vi "AlliGator Format Script Output.vi"(8 "Error In":errorcluster, 11 "Array of Simulation Outputs":T1[](array[typedef]) {"Simulation & Fit Options & Parameters"."Decay Fit Options & Parameters"."Fit Options"."Confidence Level" min=0.0 max=100.0; "Simulation & Fit Options & Parameters"."Decay Fit Options & Parameters"."Fit Options"."Offset Resolution" min=0.0; "Simulation & Fit Options & Parameters"."Decay Fit Options & Parameters"."Fit Options"."Period" min=0.0; "Simulation & Fit Options & Parameters"."Decay Fit Options & Parameters"."Fit Options"."Min Decay Percentile" min=0.0 max=1.0; "Simulation & Fit Options & Parameters"."Decay Fit Options & Parameters"."Fit Options"."Max Decay Percentile" min=0.0 max=100.0; "Simulation & Fit Options & Parameters"."Decay Fit Options & Parameters"."Fit Parameter Constraints"."Max Value" format="%#.3g"; "Simulation & Fit Options & Parameters"."Decay Fit Options & Parameters"."Fit Parameter Constraints"."Min Value" format="%#.3g"}) -> (0 "Error Out":errorcluster, 3 "Simulation Output String":string)   [LabVIEW 2021, in "AlliGator Fit Method Benchmark.lvlib"]
uses:
  AlliGator Fit Method Benchmark.lvlib
  AlliGator FMB Output.ctl
  AlliGator Simulation & Fit Options & Parameters.ctl
  AlliGator Simulation Parameters.ctl
  AlliGator Decay Simulation Parameters.ctl
  AlliGator Fit Simulation Parameters.ctl
  Decay Fit Parameter Map/AlliGator Decay Fit Options & Parameters v3.ctl
  Fits/IRF(X)PSED/Decay Fit Options v3.ctl
  Fits/Decay Convolution/Decay Model.ctl
  Fits/Residual Type.ctl
  Fits/IRF(X)PSED/Fit Weights Type.ctl
  Fits/Non-linear Fitting Method v2.ctl
  Fits/Fit Calculation Method.ctl
  Fits/Non-linear Fitting Algorithm.ctl
  Decay Analysis/Decay Fit/AlliGator Decay Fit Parameter Constraints 2.ctl
  Fits/IRF(X)PSED/Decay Fit Parameters In List.ctl
  Fits/IRF(X)PSED/MLE Baseline Offset Type.ctl
  Arrays/Array Statistics.ctl
  Arrays/Arrays.lvlib
  Fits/Fits.lvlib
  Decay Analysis/Decay Fit/AlliGator Decay Fit.lvlib
  Decay Fit Parameter Map/AlliGator Decay Fit Parameter Map.lvlib
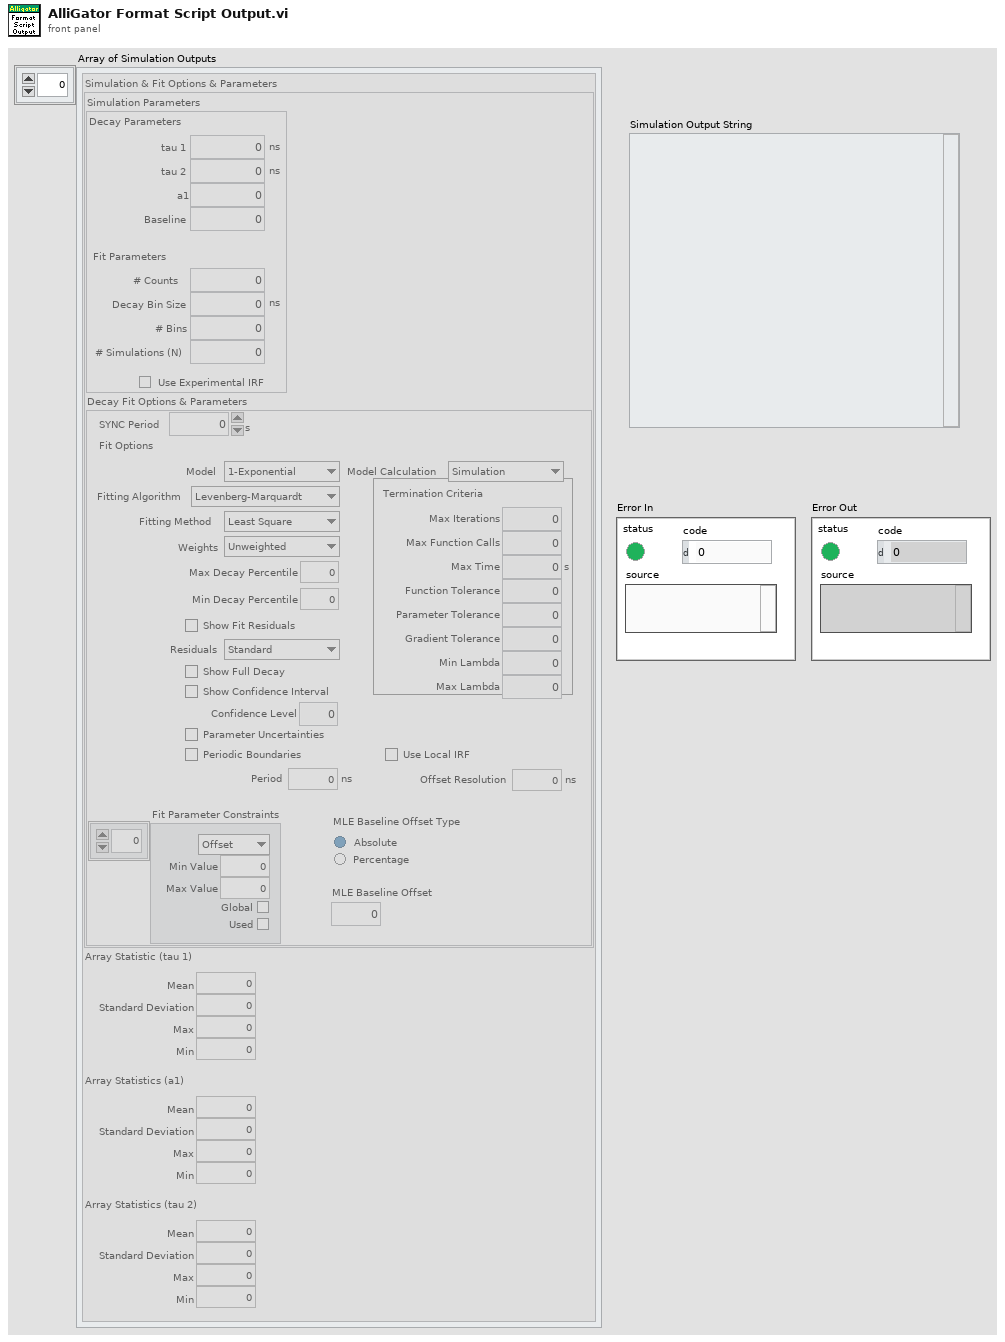
[diagram p1: front panel]
types:
  T1 = typedef "AlliGator Fit Method Benchmark.lvlib/AlliGator FMB Output.ctl" = cluster{"Simulation & Fit Options & Parameters":T2, "Array Statistic (tau 1)":T17, "Array Statistics (a1)":T17, "Array Statistics (tau 2)":T17}
  T2 = typedef "AlliGator Fit Method Benchmark.lvlib/AlliGator Simulation & Fit Options & Parameters.ctl" = cluster{"Simulation Parameters":T3, "Decay Fit Options & Parameters":T6}
  T3 = typedef "AlliGator Fit Method Benchmark.lvlib/AlliGator Simulation Parameters.ctl" = cluster{"Decay Simulation Parameters":T4, "Fit Simulation Parameters":T5, "Use Experimental IRF":bool}
  T4 = typedef "AlliGator Fit Method Benchmark.lvlib/AlliGator Decay Simulation Parameters.ctl" = cluster{"tau 1":dbl[unit], "tau 2":dbl[unit], "a1":dbl, "Baseline":dbl}
  T5 = typedef "AlliGator Fit Method Benchmark.lvlib/AlliGator Fit Simulation Parameters.ctl" = cluster{"# Counts":i32, "# Simulations (N)":i32, "Decay Bin Size":dbl[unit], "# Bins":i32}
  T6 = typedef "AlliGator Decay Fit Parameter Map.lvlib/AlliGator Decay Fit Options & Parameters v3.ctl" = cluster{"SYNC Period":dbl[unit], "Fit Options":T7, "Fit Parameter Constraints":T14[], "MLE Baseline Offset":dbl, "MLE Baseline Offset Type":T16}
  T7 = typedef "Fits.lvlib/Decay Fit Options v3.ctl" = cluster{"Show Fit Residuals":bool, "Fit Model":T8, "Residual Type":T9, "Max Decay Percentile":dbl, "Min Decay Percentile":dbl, "Show Full Decay":bool, "Weights":T10, "Fitting Method":T11, "Compute Parameter Uncertainties":bool, "Periodic Boundaries":bool, "Model Calculation":T12, "Period":dbl[unit], "Termination Criteria":cluster{"Max Iterations":i32, "Max Function Calls":i32, "Max Time":dbl[unit], "Function Tolerance":dbl, "Parameter Tolerance":dbl, "Gradient Tolerance":dbl, "Min Lambda":dbl, "Max Lambda":dbl, "Initial Tick Count":u32}, "Offset Resolution":dbl[unit], "Use Local IRF":bool, "Fitting Algorithm":T13, "Show Confidence Interval ":bool, "Confidence Level":dbl}
  T8 = typedef "Fits.lvlib/Decay Model.ctl" = enum16{"1-Exponential", "2-Exponentials"}
  T9 = typedef "Fits.lvlib/Residual Type.ctl" = enum16{"Standard", "Normalized", "Reduced"}
  T10 = typedef "Fits.lvlib/Fit Weights Type.ctl" = enum16{"Unweighted", "1/Variance", "Best of All"}
  T11 = typedef "Fits.lvlib/Non-linear Fitting Method v2.ctl" = enum16{"Least Square", "Least Absolute Residual", "Bisquare", "MLE", "-", "Best of All"}
  T12 = typedef "Fits.lvlib/Fit Calculation Method.ctl" = enum16{"Simulation", "Convolution", "Integration"}
  T13 = typedef "Fits.lvlib/Non-linear Fitting Algorithm.ctl" = enum16{"Levenberg-Marquardt", "Trust-Region Dogleg"}
  T14 = typedef "AlliGator Decay Fit.lvlib/AlliGator Decay Fit Parameter Constraints 2.ctl" = cluster{"Fit Parameter":T15, "Min Value":dbl, "Max Value":dbl, "Global":bool, "Used":bool}
  T15 = typedef "Fits.lvlib/Decay Fit Parameters In List.ctl" = enum16{"Offset", "Baseline", "A_1", "tau_1", "A_2", "tau_2"}
  T16 = typedef "Fits.lvlib/MLE Baseline Offset Type.ctl" = enum32{"Absolute", "Percentage"}
  T17 = typedef "Arrays.lvlib/Array Statistics.ctl" = cluster{"Mean":dbl, "Standard Deviation":dbl, "Max":dbl, "Min":dbl}
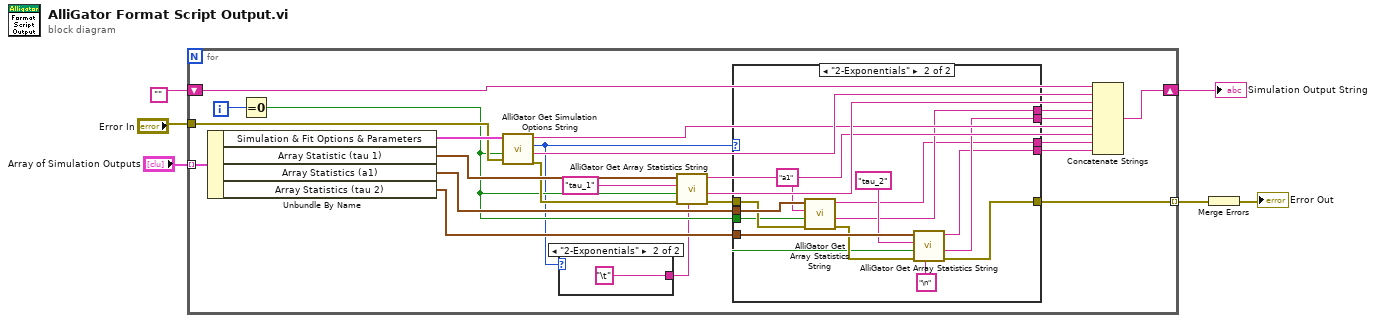
[diagram p0: block diagram]
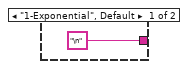
[diagram p2: hidden frame]
diagram:
  n1 = for {
    tunnel: "Array of Simulation Outputs" -> [w30] mode=indexing
    tunnel: "Error In" -> [w21]
    tunnel: [w20] -> w4 mode=indexing
    shift-right: [w18] -> w2
    shift-left: "" -> [w19]
    i -> [w24]
    n2 = Unbundle By Name(w30) -> ("Simulation & Fit Options & Parameters"=w29:T2, "Array Statistic (tau 1)"=w28:T17, "Array Statistics (a1)"=w27:T17, "Array Statistics (tau 2)"=w26:T17)
    n3 = Equal To 0?(x=w24) -> (x = 0?=w9:bool)
    n4 = call "AlliGator Get Simulation Options String.vi"("Error In"=w21, "Header Output"=w9, "Simulation & Fit Options & Parameters"=w29) -> ("Error Out"=w25:errorcluster, "Simulation Output Header String"=w17:string, "Fit Model"=w8:T8, "Simulation Output String"=w13:string)  [unwired: 5 in]
    n5 = case shown="\"2-Exponentials\"" w8 {
      tunnel: ["\n" ("End String with (\\t)") "\t" ("End String with (\\t)")] -> w7
      frame "1-Exponential", Default {
      }
      frame "2-Exponentials" {
      }
    }
    n6 = call "AlliGator Get Array Statistics String.vi"("End String with (\\t)"=w7, "Error In"=w25, "Header Output"=w9, "Array Name"="tau_1", "Array Statistic"=w28) -> ("Error Out"=w23:errorcluster, "Array Statistics Header String"=w16:string, "Array Statistics String"=w12:string)  [unwired: 4 in]
    n7 = case shown="\"2-Exponentials\"" w8 {
      tunnel: w27 -> [_ w46]
      tunnel: w26 -> [_ w45]
      tunnel: w23 -> [w33 w44]
      tunnel: [w33 w40] -> w20
      tunnel: [_ w39] -> w15
      tunnel: [_ w38] -> w14
      tunnel: [_ w36] -> w11
      tunnel: [_ w35] -> w10
      tunnel: w9 -> [_ w34]
      frame "1-Exponential", Default {
      }
      frame "2-Exponentials" {
        n8 = call "AlliGator Get Array Statistics String.vi"("Error In"=w44, "Header Output"=w34, "Array Name"="a1", "Array Statistic"=w46) -> ("Error Out"=w43:errorcluster, "Array Statistics Header String"=w39:string, "Array Statistics String"=w36:string)  [unwired: 5 in]
        n9 = call "AlliGator Get Array Statistics String.vi"("End String with (\\t)"="\n" ("End String with (\\t)"), "Error In"=w43, "Header Output"=w34, "Array Name"="tau_2", "Array Statistic"=w45) -> ("Error Out"=w40:errorcluster, "Array Statistics Header String"=w38:string, "Array Statistics String"=w35:string)  [unwired: 4 in]
      }
    }
    n10 = Concatenate Strings(w19, w17, w16, w15, w14, w13, w12, w11, w10) -> (w18:string)
  }
  "Simulation Output String" <- w2
  n11 = Merge Errors(w4) -> (→"Error Out":errorcluster)
